vi "Modify icon editor project to deploy to LVAddons.vi"(3 "Exit code":i32, 11 "Arguments":string[](array[string])) -> (2 "Output error":string)   [LabVIEW 2021]
panel:
  out "error out":errorcluster
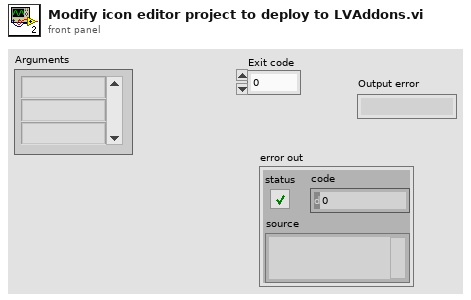
[diagram p1: front panel]
types:
  T1 = enum16{"open", "replace", "create", "open or create", "replace or create", "replace or create with confirmation"}
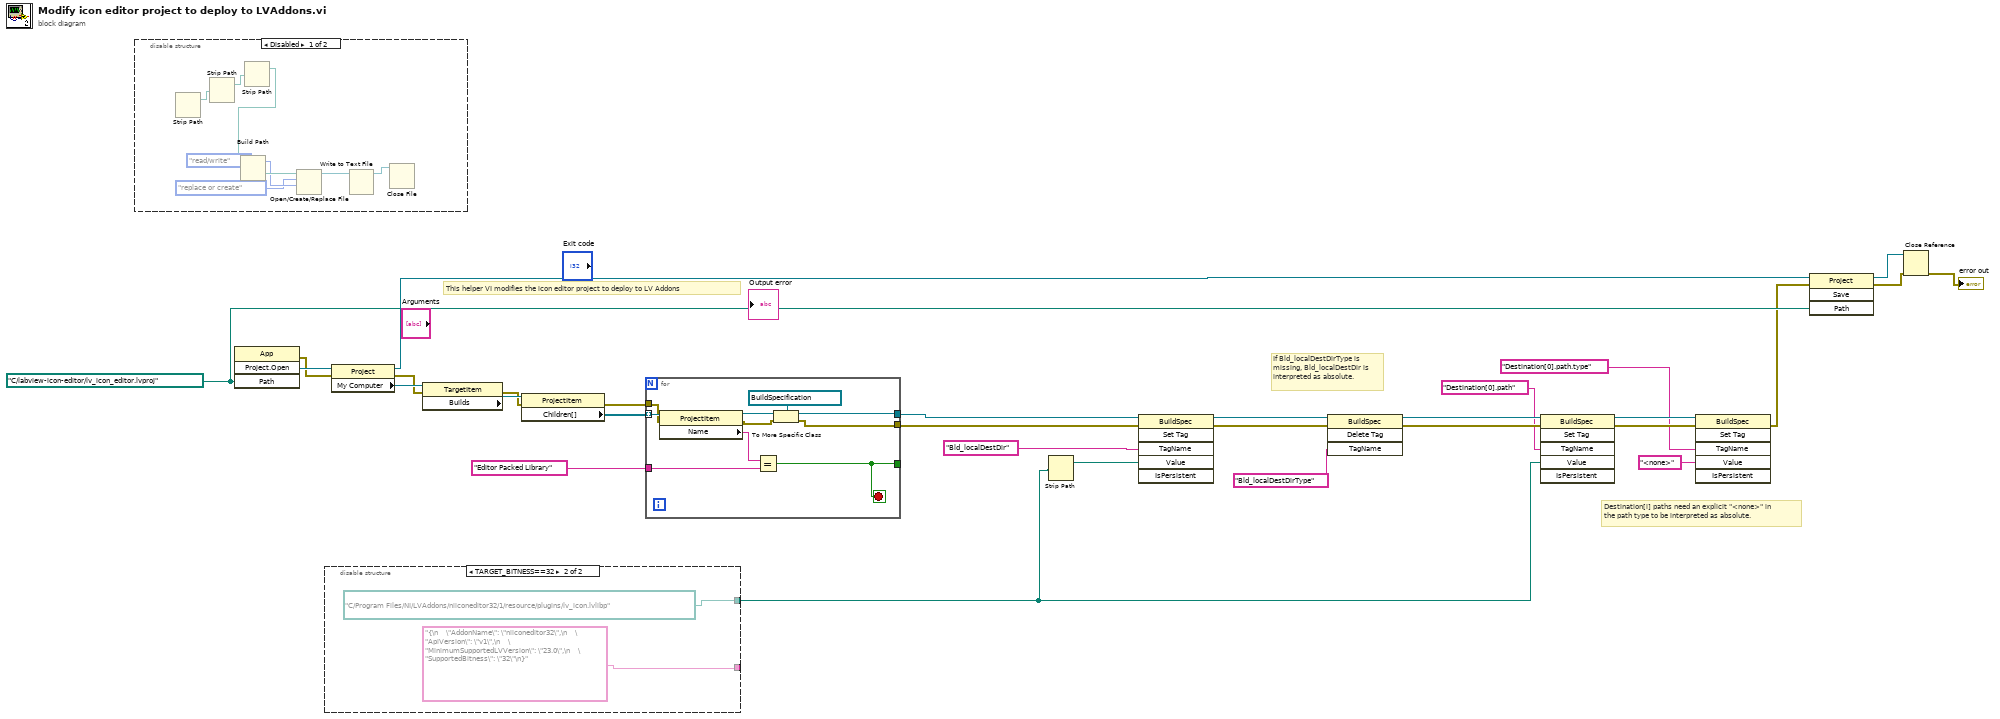
[diagram p0: block diagram]
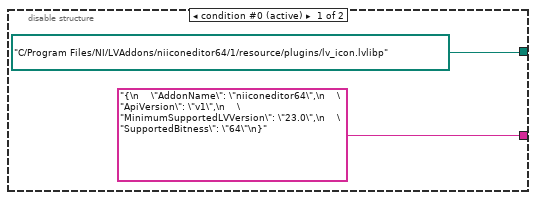
[diagram p2: hidden frame]
diagram:
  w22 = path "C:/labview-icon-editor/lv_icon_editor.lvproj" ("Path to project")
  # "Destination[i] paths need an explicit \"<none>\" in the path type to be interpreted as absolute."
  # "If Bld_localDestDirType is missing, Bld_localDestDir is interpreted as absolute."
  # "This helper VI modifies the icon editor project to deploy to LV Addons"
  n1 = disable-structure shown="Disabled" {
    frame Disabled {
      n2 = Strip Path() -> (stripped path=w36:path)  [unwired: 1 in, 1 out]
      n3 = Strip Path(path=w36) -> (stripped path=w35:path)  [unwired: 1 out]
      n4 = Strip Path(path=w35) -> (stripped path=w37:path)  [unwired: 1 out]
      n5 = Build Path(base path=w37) -> (appended path=w33:path)  [unwired: 1 in]
      n6 = Open/Create/Replace File(file path (use dialog)=w33, operation (0:open)=T1."replace or create", access (0:read/write)=enum16{"read/write", "read-only", "write-only"}."read/write") -> (refnum out=w34:refnum<file>)  [unwired: 3 in, 2 out]
      n7 = Write to Text File(file (use dialog)=w34) -> (refnum out=w38:refnum<file>)  [unwired: 3 in, 2 out]
      n8 = Close File(refnum=w38) -> ()  [unwired: 1 in, 2 out]
    }
    frame Enabled {
    }
  }
  n9 = invoke class="App" method="Project.Open"("Path"=w22) -> (error out=w8:errorcluster, "Project:Open"=w24:refnum<vi>)  [unwired: 3 in, 2 out]
  n10 = disable-structure shown="TARGET_BITNESS==32" {
    disable-tunnel: [path "C:/Program Files/NI/LVAddons/niiconeditor64/1/resource/plugins/lv_icon.lvlibp" ("Destination[i] Paths (Absolute)") path "C:/Program Files/NI/LVAddons/niiconeditor32/1/resource/plugins/lv_icon.lvlibp" ("Destination[i] Paths (Absolute)")] -> w5
    disable-tunnel: ["{\n    \"AddonName\": \"niiconeditor64\",\n    \"ApiVersion\": \"v1\",\n    \"MinimumSupportedLVVersion\": \"23.0\",\n    \"SupportedBitness\": \"64\"\n}" ("Tag Name") "{\n    \"AddonName\": \"niiconeditor32\",\n    \"ApiVersion\": \"v1\",\n    \"MinimumSupportedLVVersion\": \"23.0\",\n    \"SupportedBitness\": \"32\"\n}" ("Tag Name")] -> _
    frame condition #0 (active) {
    }
    frame condition #1 {
    }
  }
  n11 = property class="Project"(reference=w24, error in=w8) -> (reference out=w23:refnum<vi>, error out=w7:errorcluster, "My Computer"=w30:refnum<vi>)
  n12 = property class="TargetItem"(reference=w30, error in=w7) -> (error out=w6:errorcluster, "Builds"=w27:refnum<vi>)  [unwired: 1 out]
  n13 = property class="ProjectItem"(reference=w27, error in=w6) -> (error out=w4:errorcluster, "Children[]"=w29:refnum<vi>[])  [unwired: 1 out]
  n14 = for {
    tunnel: w29 -> [w52] mode=indexing
    tunnel: [w45] -> w26
    tunnel: "Editor Packed Library" ("y") -> [w50]
    tunnel: [w49] -> _
    tunnel: [w46] -> w25
    tunnel: w4 -> [w43]
    stop <- w49 stop-if-true
    n15 = property class="ProjectItem"(reference=w52, error in=w43) -> (reference out=w47:refnum<vi>, error out=w48:errorcluster, "Name"=w51:string)
    n16 = Equal?(x=w51, y=w50) -> (x = y?=w49:bool)
    n17 = To More Specific Class(target class=refnum<vi> refnum ("Build Spec"), reference=w47, error in=w48) -> (specific class reference=w45:refnum<vi>, error out=w46:errorcluster)
  }
  n18 = Strip Path(path=w5) -> (stripped path=w9:path)  [unwired: 1 out]
  n19 = invoke class="BuildSpec" method="Set Tag"(reference=w26, error in=w25, "TagName"="Bld_localDestDir" ("Tag Name"), "Value"=w9) -> (reference out=w21:refnum<vi>, error out=w17:errorcluster)  [unwired: 2 in, 4 out]
  n20 = invoke class="BuildSpec" method="Delete Tag"(reference=w21, error in=w17, "TagName"="Bld_localDestDirType" ("Tag Name")) -> (reference out=w20:refnum<vi>, error out=w16:errorcluster)  [unwired: 1 in, 2 out]
  n21 = invoke class="BuildSpec" method="Set Tag"(reference=w20, error in=w16, "TagName"="Destination[0].path" ("format string"), "Value"=w5) -> (reference out=w15:refnum<vi>, error out=w14:errorcluster)  [unwired: 2 in, 4 out]
  n22 = invoke class="BuildSpec" method="Set Tag"(reference=w15, error in=w14, "TagName"="Destination[0].path.type" ("format string"), "Value"="<none>") -> (error out=w10:errorcluster)  [unwired: 2 in, 5 out]
  n23 = invoke class="Project" method="Save"(reference=w23, error in=w10, "Path"=w22) -> (reference out=w1:refnum<vi>, error out=w3:errorcluster)  [unwired: 1 in, 2 out]
  n24 = Close Reference(reference=w1, error in (no error)=w3) -> (error out=→"error out":errorcluster)
